vi "手势获取(主).vi"() -> ()   [LabVIEW 2014]
uses:
  <vilib>/userdefined/High Color/IMAQdx.ctl
  <vilib>/vision/driver/NI_Vision_Acquisition_Software.lvlib
  <vilib>/vision/NI_Vision_Development_Module.lvlib
panel:
  out "布尔":bool
  out "操作员":string
  in  "停止":bool
  in  "选项卡控件":enum32{"用户登录", "获取手势模板", "手势匹配", "保存手势模板"}(tab)
  in  "OK":bool
  in  "登录名":string
  in  "密码":string
  in  "确定按钮":bool
  out "下":T1(plugin-control)
  in  "相机选择":T2="cam0"
  out "获取模板":T1(plugin-control)
  out "左":T1(plugin-control)
  out "上":T1(plugin-control)
  out "右":T1(plugin-control)
  in  "手势选择":enum16{"上", "下", "左", "右"}(ring)
  in  "确定按钮 2":bool
  out "下1":bool
  out "左1":bool
  out "上1":bool
  out "失败":bool
  out "右1":bool
  out "获取手势":T1(plugin-control)
  in  "上匹配算法":i32(ring)=2 items=["All", "Low Discrepancy Sampling", "Grayscale Value Pyramid", "Gradients Pyramid"]
  in  "下匹配算法":i32(ring)=2 items=["All", "Low Discrepancy Sampling", "Grayscale Value Pyramid", "Gradients Pyramid"]
  in  "左匹配算法":i32(ring)=2 items=["All", "Low Discrepancy Sampling", "Grayscale Value Pyramid", "Gradients Pyramid"]
  in  "匹配算法右":i32(ring)=2 items=["All", "Low Discrepancy Sampling", "Grayscale Value Pyramid", "Gradients Pyramid"]
  in  "上匹配参数":T3={"Number of Matches Requested"=1, "上匹配度"=500.0, "Angle Ranges"=[]} {"Angle Ranges"."End Angle" min=-360 max=360; "Angle Ranges"."Start Angle" min=-360 max=360; "上匹配度" min=0 max=1000; "Number of Matches Requested" min=1 max=9999}
  in  "下匹配参数":T4={"Number of Matches Requested"=1, "下匹配度"=500.0, "Angle Ranges"=[]} {"Angle Ranges"."End Angle" min=-360 max=360; "Angle Ranges"."Start Angle" min=-360 max=360; "下匹配度" min=0 max=1000; "Number of Matches Requested" min=1 max=9999}
  in  "右匹配参数":T5={"Number of Matches Requested"=1, "右匹配度"=500.0, "Angle Ranges"=[]} {"Angle Ranges"."End Angle" min=-360 max=360; "Angle Ranges"."Start Angle" min=-360 max=360; "右匹配度" min=0 max=1000; "Number of Matches Requested" min=1 max=9999}
  in  "左匹配参数":T6={"Number of Matches Requested"=1, "左匹配度"=500.0, "Angle Ranges"=[]} {"Angle Ranges"."End Angle" min=-360 max=360; "Angle Ranges"."Start Angle" min=-360 max=360; "左匹配度" min=0 max=1000; "Number of Matches Requested" min=1 max=9999}
  out "上2":T1(plugin-control)
  out "下2":T1(plugin-control)
  out "左2":T1(plugin-control)
  out "右2":T1(plugin-control)
  in  "开始识别":bool
  in  "最小匹配度":sgl=500.0
  in  "保存":bool
  out "右0":T1(plugin-control)
  out "左0":T1(plugin-control)
  out "下0":T1(plugin-control)
  out "上0":T1(plugin-control)
  in  "保存路径":path
  out "右模板信息":T7={"Template Contrast"=0, "Grayvalue Max Pyramid Level"=-1, "Grayvalue Optimal Pyramid Level"=-1, "Gradient Max Pyramid Level"=-1, "Gradient Optimal Pyramid Level"=-1}
  out "左模板信息":T7={"Template Contrast"=0, "Grayvalue Max Pyramid Level"=-1, "Grayvalue Optimal Pyramid Level"=-1, "Gradient Max Pyramid Level"=-1, "Gradient Optimal Pyramid Level"=-1}
  out "下模板信息":T7={"Template Contrast"=0, "Grayvalue Max Pyramid Level"=-1, "Grayvalue Optimal Pyramid Level"=-1, "Gradient Max Pyramid Level"=-1, "Gradient Optimal Pyramid Level"=-1}
  out "上模板信息":T7={"Template Contrast"=0, "Grayvalue Max Pyramid Level"=-1, "Grayvalue Optimal Pyramid Level"=-1, "Gradient Max Pyramid Level"=-1, "Gradient Optimal Pyramid Level"=-1}
  # "结果"
  # "匹\n配\n参\n数"
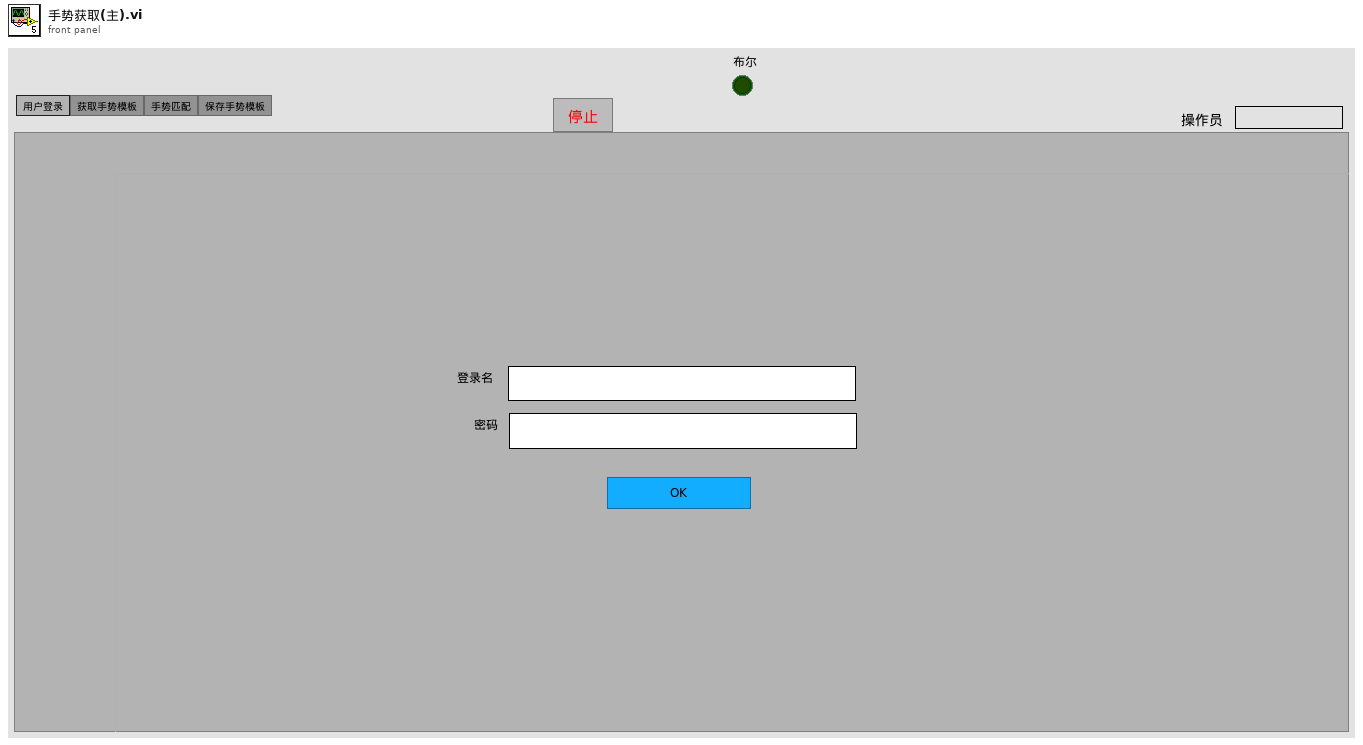
[diagram p1: front panel]
types:
  T1 = typedef "IMAQ Image.ctl" = refnum<image>
  T2 = typedef "IMAQdx.ctl" = refnum<k21>
  T3 = cluster{"Number of Matches Requested":i32, "上匹配度":sgl, "Angle Ranges":cluster{"Start Angle":sgl, "End Angle":sgl}[]}
  T4 = cluster{"Number of Matches Requested":i32, "下匹配度":sgl, "Angle Ranges":cluster{"Start Angle":sgl, "End Angle":sgl}[]}
  T5 = cluster{"Number of Matches Requested":i32, "右匹配度":sgl, "Angle Ranges":cluster{"Start Angle":sgl, "End Angle":sgl}[]}
  T6 = cluster{"Number of Matches Requested":i32, "左匹配度":sgl, "Angle Ranges":cluster{"Start Angle":sgl, "End Angle":sgl}[]}
  T7 = cluster{"Template Contrast":i32, "Grayvalue Max Pyramid Level":i32, "Grayvalue Optimal Pyramid Level":i32, "Gradient Max Pyramid Level":i32, "Gradient Optimal Pyramid Level":i32}
  T8 = typedef "Image Type" = u32
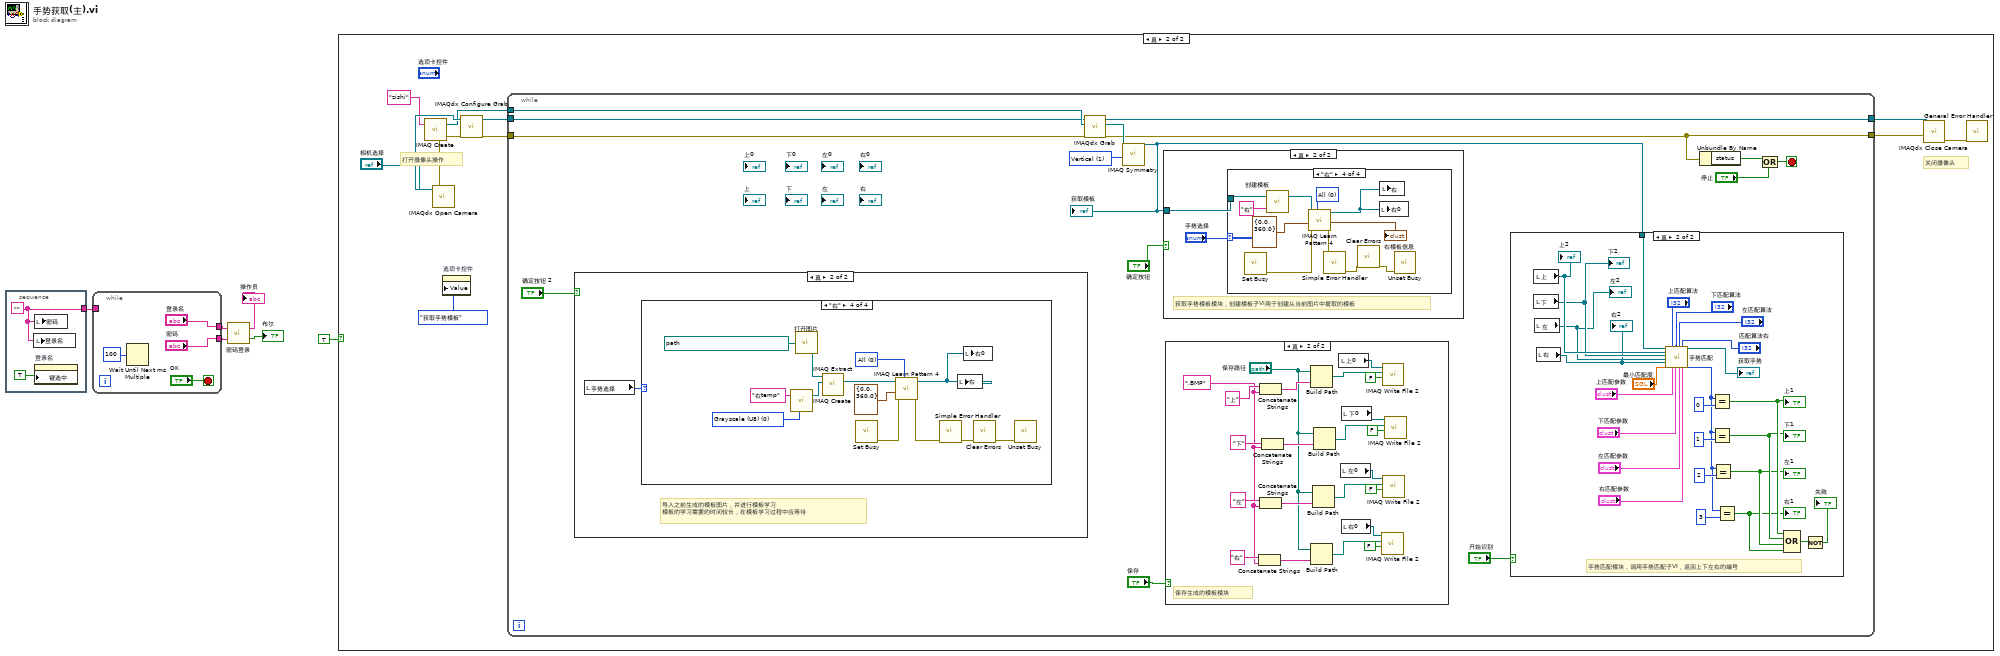
[diagram p0: block diagram]
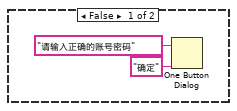
[diagram p2: hidden frame]
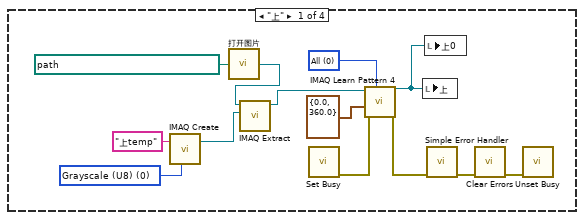
[diagram p4: hidden frame]
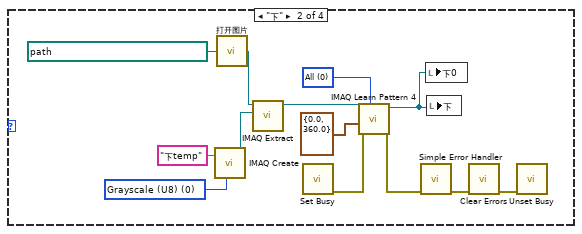
[diagram p5: hidden frame]
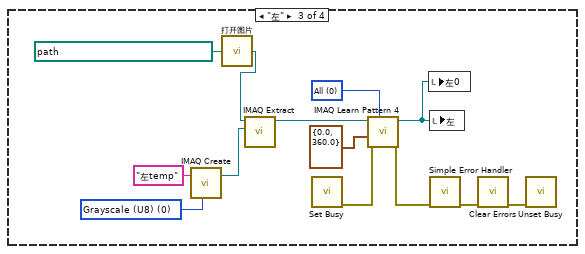
[diagram p6: hidden frame]
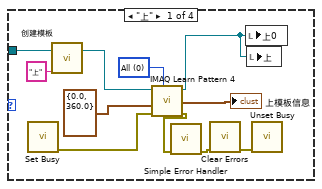
[diagram p9: hidden frame]
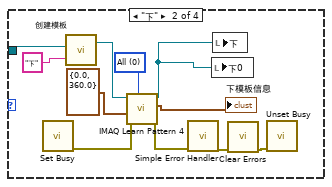
[diagram p10: hidden frame]
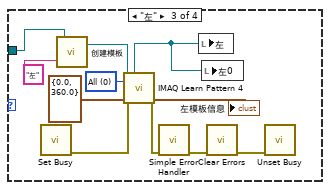
[diagram p11: hidden frame]
diagram:
  n1 = stacked-sequence {
    tunnel: [w7] -> w6
    frame #0 {
      w7 = ""
      n2 = local write "登录名"(w7) -> ()
      n3 = local write "密码"(w7) -> ()
      n4 = property on="登录名" class="Str"("键选中"=TRUE ("Key Focus")) -> ()  [unwired: 2 in, 2 out]
    }
  }
  n5 = while {
    tunnel: ["密码"] -> w3
    tunnel: ["登录名"] -> w4
    tunnel: w6 -> [_]
    stop <- "OK" stop-if-true
    n6 = Wait Until Next ms Multiple(millisecond multiple=u32 100) -> ()  [unwired: 1 out]
  }
  n7 = call "密码登录.vi"("Password"=w3, "Name"=w4) -> ("Verified"=→"布尔":bool, "Name Confirmed"=→"操作员":string)
  n8 = case shown="真" TRUE {
    frame False {
      n9 = One Button Dialog(message="请输入正确的账号密码" ("消息"), button name ("OK")="确定" ("按钮名称（“确定”）")) -> ()  [unwired: 1 out]
    }
    frame True {
      # "关闭摄像头"
      # "打开摄像头操作"
      n10 = call <vilib>:"IMAQdx Open Camera.vi"("Session In"="相机选择") -> ("error out"=w19:errorcluster, "Session Out"=w25:T2)  [unwired: 9 in]
      n11 = call "IMAQ Create"("Image Name"="zishi", "error in (no error)"=w19) -> ("New Image"=w20:T1, "error out"=w18:errorcluster)  [unwired: 3 in]
      n12 = property on="选项卡控件" class="TabCtl (严格)"("Value"=enum32{"用户登录", "获取手势模板", "手势匹配", "保存手势模板"}."获取手势模板" ("选项卡控件")) -> ()  [unwired: 2 in, 2 out]
      n13 = call <vilib>:"IMAQdx Configure Grab.vi"("error in"=w18, "Session In"=w25) -> ("error out"=w17:errorcluster, "Session Out"=w22:T2)  [unwired: 8 in]
      n14 = while {
        tunnel: w20 -> [w41]
        tunnel: w22 -> [w40]
        tunnel: [w38] -> w21
        tunnel: w17 -> [w39]
        tunnel: [w34] -> w16
        stop <- w32 stop-if-true
        w36 = u32 1 items=["Horizontal", "Vertical", "Central", "1st Diagonal", "2nd Diagonal"] ("Type of Symmetry")
        n15 = case shown="真" "确定按钮 2" {
          frame False {
          }
          frame True {
            # "导入之前生成的模板图片，并进行模板学习\n模板的学习需要的时间较长，在模板学习过程中应等待"
            n16 = local read "手势选择"() -> (w42:enum16{"上", "下", "左", "右"})
            n17 = case shown="\"右\"" w42 {
              frame "上" {
                w44 = T8 0 items=["Grayscale (U8)", "Grayscale (I16)", "Grayscale (SGL)", "Complex (CSG)", "RGB (U32)", "HSL (U32)", "RGB (U64)", "Grayscale (U16)"] ("Image Type")
                w54 = 0 items=["All", "Low Discrepancy Sampling", "Grayscale Value Pyramid", "Gradients Pyramid"] ("Algorithm")
                n18 = call "IMAQ Create"("Image Name"="上temp", "Image Type"=w44) -> ("New Image"=w43:T1)  [unwired: 3 in, 1 out]
                n19 = call "打开图片.vi"("原图路径"=path "C:/Users/26634/Desktop/labview图像处理资料/手势获取/模板图片/上.BMP") -> ("模板"=w46:T1)
                n20 = call "IMAQ Extract"("Image Dst"=w43, "Image Src"=w46) -> ("Image Dst Out"=w47:T1)  [unwired: 8 in, 1 out]
                n21 = call <vilib>:"Set Busy.vi"() -> ("error out"=w53:errorcluster)  [unwired: 10 in, 1 out]
                n22 = call "IMAQ Learn Pattern 4"("Algorithm"=w54, "error in (no error)"=w53, "Angle Range"=cluster{"Start Angle":sgl, "End Angle":sgl} {"Start Angle"=0.0, "End Angle"=360.0}, "Image"=w47) -> ("error out"=w52:errorcluster, "Template Image Out"=w48:T1)  [unwired: 5 in, 1 out]
                n23 = local write "上"(w48) -> ()
                n24 = local write "上0"(w48) -> ()
                n25 = call <vilib>:"Simple Error Handler.vi"("error in (no error)"=w52) -> ("error out"=w51:errorcluster)  [unwired: 4 in, 4 out]
                n26 = call <vilib>:"Clear Errors.vi"("error in (no error)"=w51) -> ("error out"=w50:errorcluster)  [unwired: 5 in, 1 out]
                n27 = call <vilib>:"Unset Busy.vi"("error in (no error)"=w50) -> ()  [unwired: 10 in, 1 out]
              }
              frame "下" {
                w57 = T8 0 items=["Grayscale (U8)", "Grayscale (I16)", "Grayscale (SGL)", "Complex (CSG)", "RGB (U32)", "HSL (U32)", "RGB (U64)", "Grayscale (U16)"] ("Image Type")
                w63 = 0 items=["All", "Low Discrepancy Sampling", "Grayscale Value Pyramid", "Gradients Pyramid"] ("Algorithm")
                n28 = call "IMAQ Create"("Image Name"="下temp", "Image Type"=w57) -> ("New Image"=w56:T1)  [unwired: 3 in, 1 out]
                n29 = call "打开图片.vi"("原图路径"=path "C:/Users/26634/Desktop/labview图像处理资料/手势获取/模板图片/下.BMP") -> ("模板"=w60:T1)
                n30 = call "IMAQ Extract"("Image Dst"=w56, "Image Src"=w60) -> ("Image Dst Out"=w59:T1)  [unwired: 8 in, 1 out]
                n31 = call <vilib>:"Set Busy.vi"() -> ("error out"=w64:errorcluster)  [unwired: 10 in, 1 out]
                n32 = call "IMAQ Learn Pattern 4"("Algorithm"=w63, "error in (no error)"=w64, "Angle Range"=cluster{"Start Angle":sgl, "End Angle":sgl} {"Start Angle"=0.0, "End Angle"=360.0}, "Image"=w59) -> ("error out"=w65:errorcluster, "Template Image Out"=w61:T1)  [unwired: 5 in, 1 out]
                n33 = call <vilib>:"Simple Error Handler.vi"("error in (no error)"=w65) -> ("error out"=w66:errorcluster)  [unwired: 4 in, 4 out]
                n34 = local write "下0"(w61) -> ()
                n35 = local write "下"(w61) -> ()
                n36 = call <vilib>:"Clear Errors.vi"("error in (no error)"=w66) -> ("error out"=w67:errorcluster)  [unwired: 5 in, 1 out]
                n37 = call <vilib>:"Unset Busy.vi"("error in (no error)"=w67) -> ()  [unwired: 10 in, 1 out]
              }
              frame "左" {
                w69 = T8 0 items=["Grayscale (U8)", "Grayscale (I16)", "Grayscale (SGL)", "Complex (CSG)", "RGB (U32)", "HSL (U32)", "RGB (U64)", "Grayscale (U16)"] ("Image Type")
                w76 = 0 items=["All", "Low Discrepancy Sampling", "Grayscale Value Pyramid", "Gradients Pyramid"] ("Algorithm")
                n38 = call "IMAQ Create"("Image Name"="左temp", "Image Type"=w69) -> ("New Image"=w70:T1)  [unwired: 3 in, 1 out]
                n39 = call "打开图片.vi"("原图路径"=path "C:/Users/26634/Desktop/labview图像处理资料/手势获取/模板图片/左.BMP") -> ("模板"=w72:T1)
                n40 = call "IMAQ Extract"("Image Dst"=w70, "Image Src"=w72) -> ("Image Dst Out"=w73:T1)  [unwired: 8 in, 1 out]
                n41 = call <vilib>:"Set Busy.vi"() -> ("error out"=w77:errorcluster)  [unwired: 10 in, 1 out]
                n42 = call "IMAQ Learn Pattern 4"("Algorithm"=w76, "error in (no error)"=w77, "Angle Range"=cluster{"Start Angle":sgl, "End Angle":sgl} {"Start Angle"=0.0, "End Angle"=360.0}, "Image"=w73) -> ("error out"=w78:errorcluster, "Template Image Out"=w74:T1)  [unwired: 5 in, 1 out]
                n43 = local write "左0"(w74) -> ()
                n44 = local write "左"(w74) -> ()
                n45 = call <vilib>:"Simple Error Handler.vi"("error in (no error)"=w78) -> ("error out"=w79:errorcluster)  [unwired: 4 in, 4 out]
                n46 = call <vilib>:"Clear Errors.vi"("error in (no error)"=w79) -> ("error out"=w80:errorcluster)  [unwired: 5 in, 1 out]
                n47 = call <vilib>:"Unset Busy.vi"("error in (no error)"=w80) -> ()  [unwired: 10 in, 1 out]
              }
              frame "右" {
                w83 = T8 0 items=["Grayscale (U8)", "Grayscale (I16)", "Grayscale (SGL)", "Complex (CSG)", "RGB (U32)", "HSL (U32)", "RGB (U64)", "Grayscale (U16)"] ("Image Type")
                w89 = 0 items=["All", "Low Discrepancy Sampling", "Grayscale Value Pyramid", "Gradients Pyramid"] ("Algorithm")
                n48 = call "IMAQ Create"("Image Name"="右temp", "Image Type"=w83) -> ("New Image"=w82:T1)  [unwired: 3 in, 1 out]
                n49 = call "打开图片.vi"("原图路径"=path "C:/Users/26634/Desktop/labview图像处理资料/手势获取/模板图片/右.BMP") -> ("模板"=w85:T1)
                n50 = call "IMAQ Extract"("Image Dst"=w82, "Image Src"=w85) -> ("Image Dst Out"=w86:T1)  [unwired: 8 in, 1 out]
                n51 = call <vilib>:"Set Busy.vi"() -> ("error out"=w90:errorcluster)  [unwired: 10 in, 1 out]
                n52 = call "IMAQ Learn Pattern 4"("Algorithm"=w89, "error in (no error)"=w90, "Angle Range"=cluster{"Start Angle":sgl, "End Angle":sgl} {"Start Angle"=0.0, "End Angle"=360.0}, "Image"=w86) -> ("error out"=w91:errorcluster, "Template Image Out"=w87:T1)  [unwired: 5 in, 1 out]
                n53 = call <vilib>:"Simple Error Handler.vi"("error in (no error)"=w91) -> ("error out"=w92:errorcluster)  [unwired: 4 in, 4 out]
                n54 = local write "右"(w87) -> ()
                n55 = local write "右0"(w87) -> ()
                n56 = call <vilib>:"Clear Errors.vi"("error in (no error)"=w92) -> ("error out"=w93:errorcluster)  [unwired: 5 in, 1 out]
                n57 = call <vilib>:"Unset Busy.vi"("error in (no error)"=w93) -> ()  [unwired: 10 in, 1 out]
              }
            }
          }
        }
        n58 = call <vilib>:"IMAQdx Grab.vi"("error in"=w39, "Image In"=w41, "Session In"=w40) -> ("error out"=w34:errorcluster, "Image Out"=w37:T1, "Session Out"=w38:T2)  [unwired: 5 in, 1 out]
        n59 = call "IMAQ Symmetry"("Type of Symmetry"=w36, "Image Src"=w37) -> ("Image Dst Out"=w28:T1)  [unwired: 3 in, 1 out]
        "获取模板" <- w28
        n60 = case shown="真" "确定按钮" {
          tunnel: w28 -> [_ w121]
          frame False {
          }
          frame True {
            # "获取手势模板模块，创建模板子VI用于创建从当前图片中提取的模板"
            n61 = case shown="\"右\"" "手势选择" {
              tunnel: w121 -> [w133 w144 w155 w165]
              frame "上" {
                w130 = 0 items=["All", "Low Discrepancy Sampling", "Grayscale Value Pyramid", "Gradients Pyramid"] ("Algorithm")
                n62 = call <vilib>:"Set Busy.vi"() -> ("error out"=w126:errorcluster)  [unwired: 10 in, 1 out]
                n63 = call "创建模板.vi"("模板图片名"="上" ("字符串"), "源图片"=w133) -> ("模板"=w131:T1)  [unwired: 1 in]
                n64 = call "IMAQ Learn Pattern 4"("Algorithm"=w130, "error in (no error)"=w126, "Angle Range"=cluster{"Start Angle":sgl, "End Angle":sgl} {"Start Angle"=0.0, "End Angle"=360.0}, "Image"=w131) -> ("error out"=w125:errorcluster, "Template Report"=→"上模板信息":T7, "Template Image Out"=w124:T1)  [unwired: 5 in]
                n65 = call <vilib>:"Simple Error Handler.vi"("error in (no error)"=w125) -> ("error out"=w128:errorcluster)  [unwired: 4 in, 4 out]
                n66 = call <vilib>:"Clear Errors.vi"("error in (no error)"=w128) -> ("error out"=w127:errorcluster)  [unwired: 5 in, 1 out]
                n67 = local write "上0"(w124) -> ()
                n68 = local write "上"(w124) -> ()
                n69 = call <vilib>:"Unset Busy.vi"("error in (no error)"=w127) -> ()  [unwired: 10 in, 1 out]
              }
              frame "下" {
                w134 = 0 items=["All", "Low Discrepancy Sampling", "Grayscale Value Pyramid", "Gradients Pyramid"] ("Algorithm")
                n70 = call <vilib>:"Set Busy.vi"() -> ("error out"=w142:errorcluster)  [unwired: 10 in, 1 out]
                n71 = call "创建模板.vi"("模板图片名"="下" ("字符串"), "源图片"=w144) -> ("模板"=w137:T1)  [unwired: 1 in]
                n72 = call "IMAQ Learn Pattern 4"("Algorithm"=w134, "error in (no error)"=w142, "Angle Range"=cluster{"Start Angle":sgl, "End Angle":sgl} {"Start Angle"=0.0, "End Angle"=360.0}, "Image"=w137) -> ("error out"=w141:errorcluster, "Template Report"=→"下模板信息":T7, "Template Image Out"=w136:T1)  [unwired: 5 in]
                n73 = call <vilib>:"Simple Error Handler.vi"("error in (no error)"=w141) -> ("error out"=w140:errorcluster)  [unwired: 4 in, 4 out]
                n74 = local write "下0"(w136) -> ()
                n75 = local write "下"(w136) -> ()
                n76 = call <vilib>:"Clear Errors.vi"("error in (no error)"=w140) -> ("error out"=w139:errorcluster)  [unwired: 5 in, 1 out]
                n77 = call <vilib>:"Unset Busy.vi"("error in (no error)"=w139) -> ()  [unwired: 10 in, 1 out]
              }
              frame "左" {
                w147 = 0 items=["All", "Low Discrepancy Sampling", "Grayscale Value Pyramid", "Gradients Pyramid"] ("Algorithm")
                n78 = call <vilib>:"Set Busy.vi"() -> ("error out"=w153:errorcluster)  [unwired: 10 in, 1 out]
                n79 = call "创建模板.vi"("模板图片名"="左" ("字符串"), "源图片"=w155) -> ("模板"=w148:T1)  [unwired: 1 in]
                n80 = call "IMAQ Learn Pattern 4"("Algorithm"=w147, "error in (no error)"=w153, "Angle Range"=cluster{"Start Angle":sgl, "End Angle":sgl} {"Start Angle"=0.0, "End Angle"=360.0}, "Image"=w148) -> ("error out"=w152:errorcluster, "Template Report"=→"左模板信息":T7, "Template Image Out"=w146:T1)  [unwired: 5 in]
                n81 = call <vilib>:"Simple Error Handler.vi"("error in (no error)"=w152) -> ("error out"=w151:errorcluster)  [unwired: 4 in, 4 out]
                n82 = local write "左"(w146) -> ()
                n83 = local write "左0"(w146) -> ()
                n84 = call <vilib>:"Clear Errors.vi"("error in (no error)"=w151) -> ("error out"=w150:errorcluster)  [unwired: 5 in, 1 out]
                n85 = call <vilib>:"Unset Busy.vi"("error in (no error)"=w150) -> ()  [unwired: 10 in, 1 out]
              }
              frame "右" {
                w164 = 0 items=["All", "Low Discrepancy Sampling", "Grayscale Value Pyramid", "Gradients Pyramid"] ("Algorithm")
                n86 = call <vilib>:"Set Busy.vi"() -> ("error out"=w163:errorcluster)  [unwired: 10 in, 1 out]
                n87 = call "创建模板.vi"("模板图片名"="右" ("字符串"), "源图片"=w165) -> ("模板"=w156:T1)  [unwired: 1 in]
                n88 = call "IMAQ Learn Pattern 4"("Algorithm"=w164, "error in (no error)"=w163, "Angle Range"=cluster{"Start Angle":sgl, "End Angle":sgl} {"Start Angle"=0.0, "End Angle"=360.0}, "Image"=w156) -> ("error out"=w162:errorcluster, "Template Report"=→"右模板信息":T7, "Template Image Out"=w157:T1)  [unwired: 5 in]
                n89 = call <vilib>:"Simple Error Handler.vi"("error in (no error)"=w162) -> ("error out"=w161:errorcluster)  [unwired: 4 in, 4 out]
                n90 = call <vilib>:"Clear Errors.vi"("error in (no error)"=w161) -> ("error out"=w160:errorcluster)  [unwired: 5 in, 1 out]
                n91 = local write "右0"(w157) -> ()
                n92 = local write "右"(w157) -> ()
                n93 = call <vilib>:"Unset Busy.vi"("error in (no error)"=w160) -> ()  [unwired: 10 in, 1 out]
              }
            }
          }
        }
        n94 = case shown="真" "保存" {
          frame False {
          }
          frame True {
            w176 = ".BMP" ("字符串")
            # "保存生成的模板模块"
            n95 = Concatenate Strings("右" ("字符串"), w176) -> (w181:string)
            n96 = Concatenate Strings("上" ("字符串"), w176) -> (w187:string)
            n97 = Concatenate Strings("左" ("字符串"), w176) -> (w182:string)
            n98 = Concatenate Strings("下" ("字符串"), w176) -> (w185:string)
            n99 = Build Path(base path="保存路径", name or relative path=w187) -> (appended path=w188:path)
            n100 = Build Path(base path="保存路径", name or relative path=w181) -> (appended path=w180:path)
            n101 = Build Path(base path="保存路径", name or relative path=w182) -> (appended path=w183:path)
            n102 = Build Path(base path="保存路径", name or relative path=w185) -> (appended path=w184:path)
            n103 = local read "上0"() -> (w174:T1)
            n104 = local read "左0"() -> (w172:T1)
            n105 = local read "右0"() -> (w171:T1)
            n106 = local read "下0"() -> (w173:T1)
            n107 = call-poly "IMAQ Write File 2"("Compress? (N)"=FALSE, "File Path"=w180, "Image"=w171) -> ()  [unwired: 7 in, 2 out]
            n108 = call-poly "IMAQ Write File 2"("Compress? (N)"=FALSE, "File Path"=w188, "Image"=w174) -> ()  [unwired: 7 in, 2 out]
            n109 = call-poly "IMAQ Write File 2"("Compress? (N)"=FALSE, "File Path"=w183, "Image"=w172) -> ()  [unwired: 7 in, 2 out]
            n110 = call-poly "IMAQ Write File 2"("Compress? (N)"=FALSE, "File Path"=w184, "Image"=w173) -> ()  [unwired: 7 in, 2 out]
          }
        }
        n111 = case shown="真" "开始识别" {
          tunnel: w28 -> [_ w100]
          frame False {
          }
          frame True {
            # "手势匹配模块，调用手势匹配子VI，返回上下左右的编号"
            n112 = local read "上"() -> (w98:T1)
            "上2" <- w98
            n113 = local read "下"() -> (w97:T1)
            "下2" <- w97
            n114 = local read "左"() -> (w96:T1)
            "左2" <- w96
            n115 = local read "右"() -> (w95:T1)
            "右2" <- w95
            n116 = call "手势匹配.vi"("源图片"=w100, "上"=w98, "下"=w97, "左"=w96, "右"=w95, "最小匹配度"="最小匹配度", "匹配算法0"="上匹配算法", "匹配参数0"="上匹配参数", "匹配算法1"="下匹配算法", "匹配参数1"="下匹配参数", "匹配算法2"="左匹配算法", "匹配参数2"="左匹配参数", "匹配算法3"="匹配算法右", "匹配参数3"="右匹配参数") -> ("输出图"=→"获取手势":T1, "结果"=w110:i32)  [unwired: 4 in]
            n117 = Equal?(x=w110, y=0) -> (x = y?=w116:bool)
            "上1" <- w116
            n118 = Equal?(x=w110, y=1) -> (x = y?=w115:bool)
            "下1" <- w115
            n119 = Equal?(x=w110, y=2) -> (x = y?=w114:bool)
            "左1" <- w114
            n120 = Equal?(x=w110, y=3) -> (x = y?=w113:bool)
            "右1" <- w113
            n121 = Compound Arithmetic op=OR(w116, w115, w114, w113) -> (w112:bool)
            n122 = Not(x=w112) -> (.not. x?=→"失败":bool)
          }
        }
        n123 = Unbundle By Name(w34) -> ("status"=w35:bool)
        n124 = Or(x=w35, y="停止") -> (x .or. y?=w32:bool)
      }
      n125 = call <vilib>:"IMAQdx Close Camera.vi"("error in"=w16, "Session In"=w21) -> ("error out"=w15:errorcluster)  [unwired: 9 in]
      n126 = call <vilib>:"General Error Handler.vi"("error in (no error)"=w15) -> ()  [unwired: 2 in, 13 out]
    }
  }
